vi "RTS TC Points.vi"(7 "Point Data":T2[](array[typedef]), 8 "Error In":errorcluster, 10 "TC Data":string[](array[string]), 11 "Input Save Array":T1[](array[typedef])) -> (0 "Error Out":errorcluster, 3 "Output Save Array":T1[](array[typedef]))   [LabVIEW 2019]
uses:
  Washer DOE/Type Definitions/DOE Data Save Modifier.ctl
  Type Definitions/RTS Point File.ctl
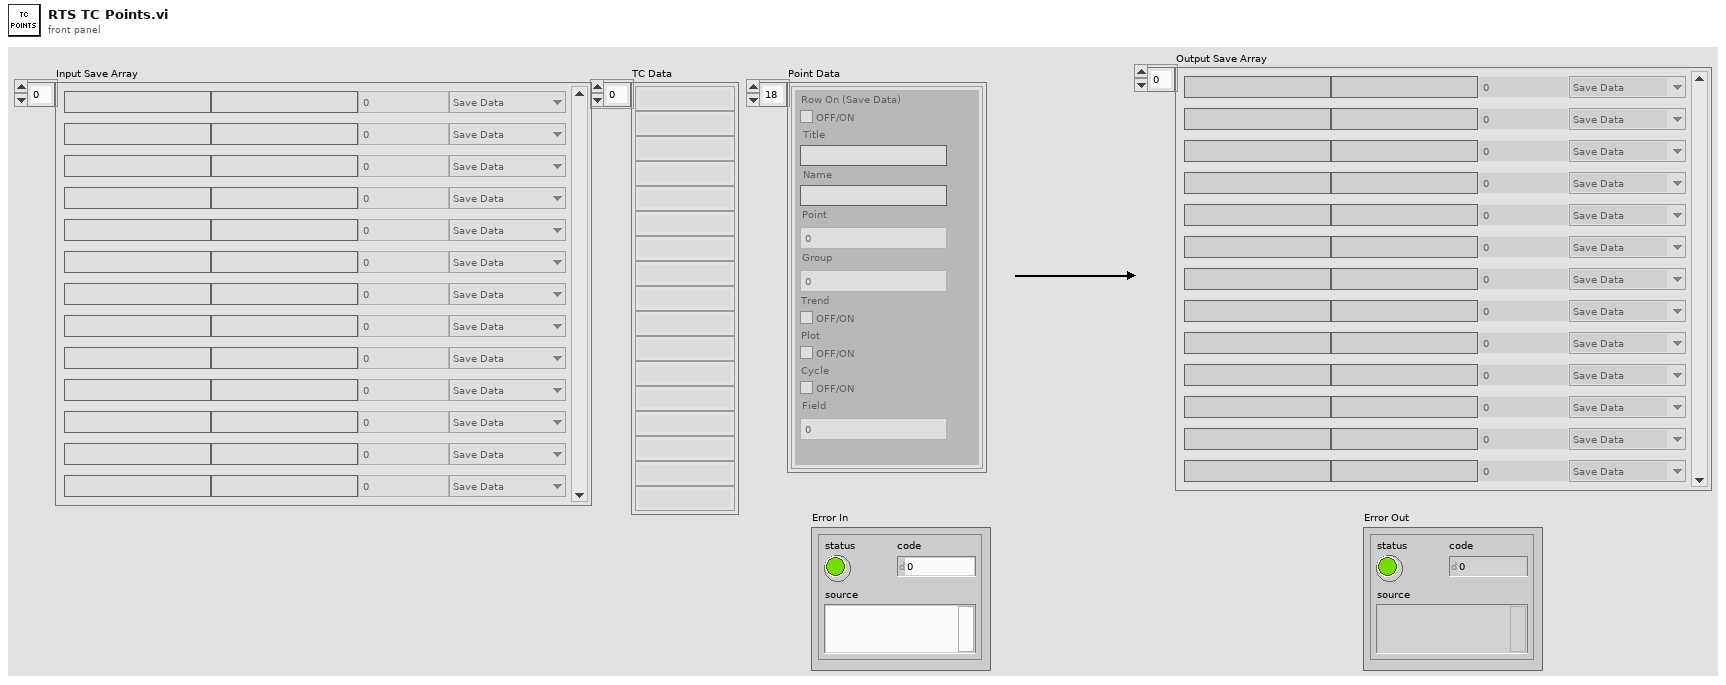
[diagram p1: front panel]
types:
  T1 = typedef "DOE Data Save Modifier.ctl" = cluster{"Name":string, "Title":string, "Save Status":enum16{"Save Data", "Don't Save Data"}, "Group":u8, "Field":u8}
  T2 = typedef "RTS Point File.ctl" = cluster{"Title":string, "Name":string, "Point":u8, "Plot":bool, "Trend":bool, "Cycle":bool, "Field":u8, "Row On (Save Data)":bool, "Group":u8}
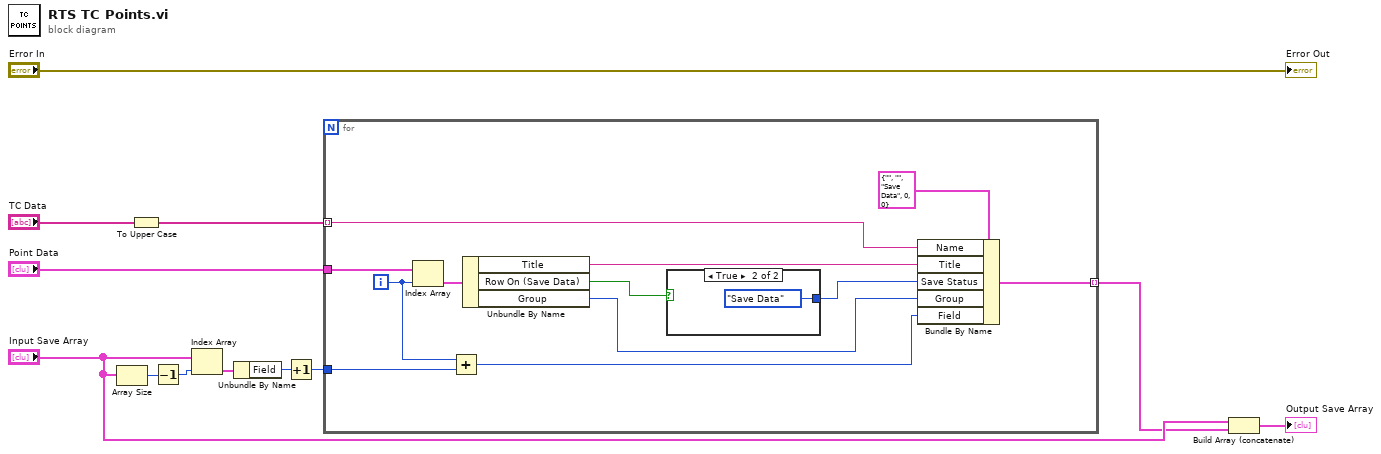
[diagram p0: block diagram]
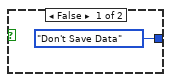
[diagram p2: hidden frame]
diagram:
  n1 = Array Size(array="Input Save Array") -> (size(s)=w9:i32)
  n2 = To Upper Case(1:"TC Data") -> (0:w1:string[])
  n3 = Decrement(x=w9) -> (x-1=w8:i32)
  n4 = Index Array(array="Input Save Array", index=w8) -> (element=w10:T1)
  n5 = Unbundle By Name(w10) -> ("Field"=w7:u8)
  n6 = Increment(x=w7) -> (x+1=w6:u8)
  n7 = for {
    tunnel: "Point Data" -> [w19]
    tunnel: [w20] -> w4 mode=indexing
    tunnel: w1 -> [w17] mode=indexing
    tunnel: w6 -> [w14]
    i -> [w15]
    n8 = Index Array(array=w19, index=w15) -> (element=w18:T2)
    n9 = Add(x=w15, y=w14) -> (x+y=w13:i32)
    n10 = Unbundle By Name(w18) -> ("Title"=w24:string, "Row On (Save Data)"=w22:bool, "Group"=w23:u8)
    n11 = case shown="True" w22 {
      tunnel: [enum16{"Save Data", "Don't Save Data"}."Don't Save Data" ("Save Status") enum16{"Save Data", "Don't Save Data"}."Save Data" ("Save Status")] -> w21
      frame False {
      }
      frame True {
      }
    }
    n12 = Bundle By Name(cluster=T1 {"Name"="", "Title"="", "Save Status"=enum."Save Data", "Group"=0, "Field"=0} ("Input Save Array"), "Name"=w17, "Title"=w24, "Save Status"=w21, "Group"=w23, "Field"=w13) -> (w20:T1)
  }
  n13 = Build Array (concatenate)("Input Save Array", w4) -> (→"Output Save Array":T1[])
  "Error Out" <- "Error In"
